vi "VI Tree.vi"   [LabVIEW 2021, in "Queue.lvlib"]
doc: "The Queue library contains the following sections:\n- <b>Examples</b>: Example VIs\n- <b>API</b>: Top-level VIs\n- <b>SubVIs</b>: Low-level VIs"
uses:
  Queue.lvlib
  16166754-5e17-4172-8fef-04d17df9ff6d.vi
  419261d6-cfd9-4367-a5e7-292623275988.vi
  b288d960-20d2-4226-b72b-ebf4ce870cf4.vi
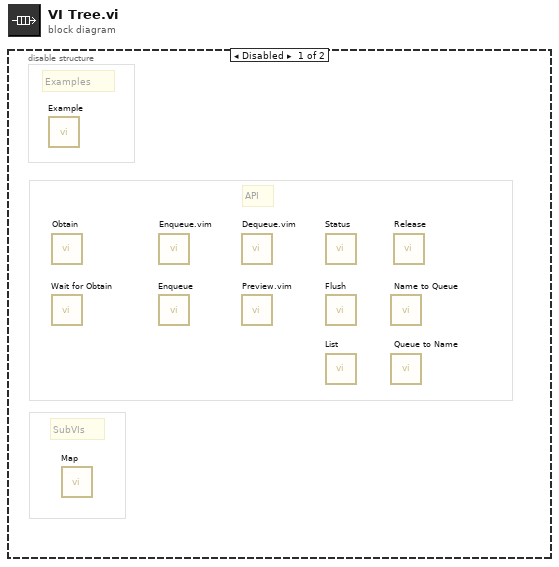
[diagram p0: block diagram]
diagram:
  n1 = disable-structure shown="Disabled" {
    frame Disabled {
      # "SubVIs"
      # "API"
      # "Examples"
      n2 = call "Example.vi"() -> ()  [unwired: 12 in]
      n3 = call "Obtain.vi"() -> ()  [unwired: 9 in, 3 out]
      n4 = call "Wait for Obtain.vi"() -> ()  [unwired: 9 in, 3 out]
      n5 = call "Map.vi"() -> ()  [unwired: 9 in, 3 out]
      n6 = call "Enqueue.vim"() -> ()  [unwired: 10 in, 2 out]
      n7 = call "Enqueue.vi"() -> ()  [unwired: 10 in, 2 out]
      n8 = call "Dequeue.vim"() -> ()  [unwired: 6 in, 6 out]
      n9 = call "Preview.vim"() -> ()  [unwired: 6 in, 6 out]
      n10 = call "Status.vi"() -> ()  [unwired: 4 in, 8 out]
      n11 = call "Flush.vi"() -> ()  [unwired: 7 in, 5 out]
      n12 = call "List.vi"() -> ()  [unwired: 9 in, 3 out]
      n13 = call "Name to Queue.vi"() -> ()  [unwired: 8 in, 2 out]
      n14 = call "Queue to Name.vi"() -> ()  [unwired: 8 in, 2 out]
      n15 = call "Release.vi"() -> ()  [unwired: 9 in, 3 out]
    }
    frame Enabled {
    }
  }
